vi "noteOnorOffEvent.vi"(10 "Volume":u8, 11 "MIDI Message":u16) -> (3 "Midi Message":u16)   [LabVIEW 2020, in "midi-ui.lvclass"]
uses:
  midi-ui.lvclass
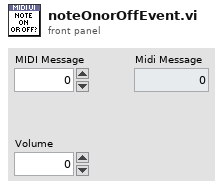
[diagram p1: front panel]
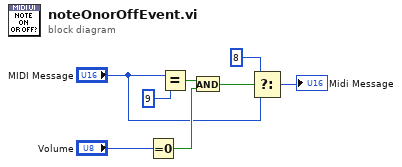
[diagram p0: block diagram]
diagram:
  n1 = Equal To 0?(x="Volume") -> (x = 0?=w6:bool)
  n2 = Equal?(x="MIDI Message", y=u16 9) -> (x = y?=w7:bool)
  n3 = And(x=w7, y=w6) -> (x .and. y?=w5:bool)
  n4 = Select(t=u16 8, s=w5, f="MIDI Message") -> (s? t:f=→"Midi Message":u16)
